vi "InitConfigutation.vi"(8 "error in":errorcluster) -> (0 "error out":errorcluster)   [LabVIEW 2013]
uses:
  <vilib>/Utility/config.llb/Read Key (U32).vi
  <vilib>/Utility/config.llb/Read Key (String).vi
  GlobalVariables/ValveParameters.vi
  GlobalVariables/CaptParameters.vi
  GlobalVariables/SystemParameters.vi
  <vilib>/Utility/config.llb/NI_LVConfig.lvlib
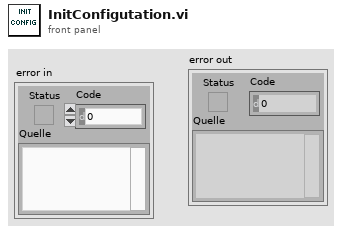
[diagram p1: front panel]
types:
  T1 = cluster{"Mode":enum16{"RTU", "ASCII"}, "Slave Address":u8}
  T2 = typedef "NI_LVConfig.lvlib/Config Data RefNum.ctl" = refnum<k1>
  T3 = cluster{"value":u32, "value":u32, "value":u32, "value":u32, "value":u32}
  T4 = cluster{"value":u32, "value":u32, "value":u32, "value":u32, "value":u32, "value":string, "Serial Parameters":cluster{"Mode":enum16{"RTU", "ASCII"}, "Slave Address":u8}, "value":u32, cluster{"value":u32, "value":u32, "value":u32, "value":u32, "value":u32}}
  T5 = cluster{"value":u32, "value":u32, "value":u32, "value":u32, "value":u32, "value":string, "value":u32, "Serial Parameters":cluster{"Mode":enum16{"RTU", "ASCII"}, "Slave Address":u8}, "value":u32}
  T6 = cluster{"value":string, "value":string, "value":string, "value":string}
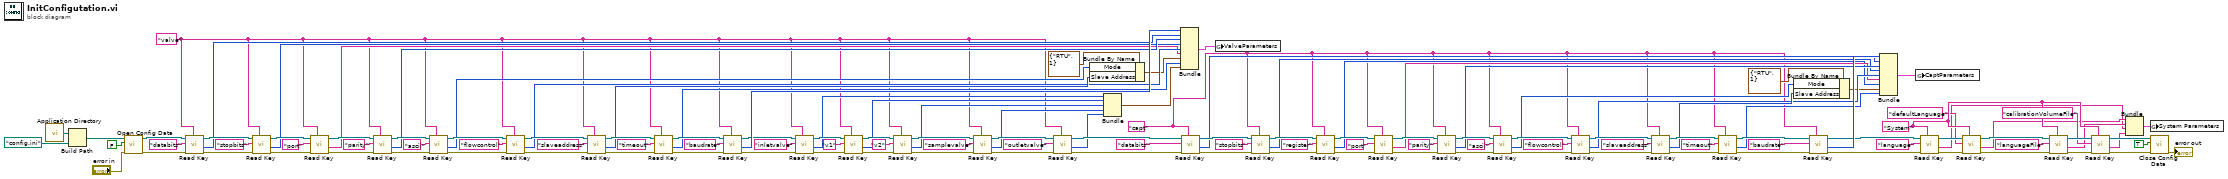
[diagram p0: block diagram]
diagram:
  w34 = "System" ("section")
  w45 = "capt" ("section")
  w6 = "valve" ("section")
  n1 = call <vilib>:"Application Directory.vi"() -> ("Application Directory"=w127:path)
  n2 = Build Path(base path=w127, name or relative path=path "config.ini" ("default name")) -> (appended path=w129:path)
  n3 = call <vilib>:"Open Config Data.vi"("error in (no error)"="error in", "create file if necessary (T)"=FALSE ("create file if necessary? (T)"), "configuration file path"=w129) -> ("error out"=w60:errorcluster, "refnum"=w59:T2)  [unwired: 6 in, 1 out]
  n4 = call-poly <vilib>:"Read Key.vi"("section"=w6, "error in (no error)"=w60, "key"="databits", "refnum"=w59) -> ("error out"=w63:errorcluster, "value"=w55:u32, "refnum out"=w62:T2)  [unwired: 4 in, 1 out]
  n5 = call-poly <vilib>:"Read Key.vi"("section"=w6, "error in (no error)"=w63, "key"="stopbits", "refnum"=w62) -> ("error out"=w61:errorcluster, "value"=w54:u32, "refnum out"=w58:T2)  [unwired: 4 in, 1 out]
  n6 = call-poly <vilib>:"Read Key.vi"("section"=w6, "error in (no error)"=w61, "key"="port", "refnum"=w58) -> ("error out"=w120:errorcluster, "value"=w100:string, "refnum out"=w119:T2)  [unwired: 4 in, 1 out]
  n7 = call-poly <vilib>:"Read Key.vi"("section"=w6, "error in (no error)"=w120, "key"="parity", "refnum"=w119) -> ("error out"=w117:errorcluster, "value"=w102:u32, "refnum out"=w114:T2)  [unwired: 4 in, 1 out]
  n8 = call-poly <vilib>:"Read Key.vi"("section"=w6, "error in (no error)"=w117, "key"="ascii", "refnum"=w114) -> ("error out"=w116:errorcluster, "value"=w107:u32, "refnum out"=w115:T2)  [unwired: 4 in, 1 out]
  n9 = call-poly <vilib>:"Read Key.vi"("section"=w6, "error in (no error)"=w116, "key"="flowcontrol", "refnum"=w115) -> ("error out"=w112:errorcluster, "value"=w101:u32, "refnum out"=w109:T2)  [unwired: 4 in, 1 out]
  n10 = call-poly <vilib>:"Read Key.vi"("section"=w6, "error in (no error)"=w112, "key"="slaveaddress", "refnum"=w109) -> ("error out"=w111:errorcluster, "value"=w106:u32, "refnum out"=w110:T2)  [unwired: 4 in, 1 out]
  n11 = call-poly <vilib>:"Read Key.vi"("section"=w6, "error in (no error)"=w111, "key"="timeout", "refnum"=w110) -> ("error out"=w124:errorcluster, "value"=w98:u32, "refnum out"=w125:T2)  [unwired: 4 in, 1 out]
  n12 = call-poly <vilib>:"Read Key.vi"("section"=w6, "error in (no error)"=w124, "key"="baudrate", "refnum"=w125) -> ("error out"=w23:errorcluster, "value"=w103:u32, "refnum out"=w13:T2)  [unwired: 4 in, 1 out]
  n13 = call-poly <vilib>:"Read Key.vi"("section"=w6, "error in (no error)"=w23, "key"="inletvalve", "refnum"=w13) -> ("error out"=w24:errorcluster, "value"=w11:u32, "refnum out"=w14:T2)  [unwired: 4 in, 1 out]
  n14 = call-poly <vilib>:"Read Key.vi"("section"=w6, "error in (no error)"=w24, "key"="v1", "refnum"=w14) -> ("error out"=w22:errorcluster, "value"=w10:u32, "refnum out"=w15:T2)  [unwired: 4 in, 1 out]
  n15 = call-poly <vilib>:"Read Key.vi"("section"=w6, "error in (no error)"=w22, "key"="v2", "refnum"=w15) -> ("error out"=w21:errorcluster, "value"=w9:u32, "refnum out"=w16:T2)  [unwired: 4 in, 1 out]
  n16 = call-poly <vilib>:"Read Key.vi"("section"=w6, "error in (no error)"=w21, "key"="samplevalve", "refnum"=w16) -> ("error out"=w20:errorcluster, "value"=w8:u32, "refnum out"=w17:T2)  [unwired: 4 in, 1 out]
  n17 = call-poly <vilib>:"Read Key.vi"("section"=w6, "error in (no error)"=w20, "key"="outletvalve", "refnum"=w17) -> ("error out"=w19:errorcluster, "value"=w7:u32, "refnum out"=w18:T2)  [unwired: 4 in, 1 out]
  n18 = Bundle By Name(cluster=T1 {"Mode"=enum."RTU", "Slave Address"=1} ("Serial Parameters"), "Mode"=w107, "Slave Address"=w106) -> (w99:T1)
  n19 = Bundle("value"=w11, "value"=w10, "value"=w9, "value"=w8, "value"=w7) -> (w12:T3)  [unwired: 1 in]
  n20 = Bundle("value"=w103, "value"=w55, "value"=w102, "value"=w54, "value"=w101, "value"=w100, "Serial Parameters"=w99, "value"=w98, w12) -> (w104:T4)  [unwired: 1 in]
  n21 = call-poly <vilib>:"Read Key.vi"("section"=w45, "error in (no error)"=w19, "key"="databits", "refnum"=w18) -> ("error out"=w53:errorcluster, "value"=w47:u32, "refnum out"=w52:T2)  [unwired: 4 in, 1 out]
  n22 = global write "ValveParameters.vi" "ValveParameters"(w104) -> ()
  n23 = call-poly <vilib>:"Read Key.vi"("section"=w45, "error in (no error)"=w53, "key"="stopbits", "refnum"=w52) -> ("error out"=w48:errorcluster, "value"=w46:u32, "refnum out"=w49:T2)  [unwired: 4 in, 1 out]
  n24 = call-poly <vilib>:"Read Key.vi"("section"=w45, "error in (no error)"=w48, "key"="register", "refnum"=w49) -> ("error out"=w67:errorcluster, "value"=w65:u32, "refnum out"=w66:T2)  [unwired: 4 in, 1 out]
  n25 = call-poly <vilib>:"Read Key.vi"("section"=w45, "error in (no error)"=w67, "key"="port", "refnum"=w66) -> ("error out"=w91:errorcluster, "value"=w72:string, "refnum out"=w90:T2)  [unwired: 4 in, 1 out]
  n26 = call-poly <vilib>:"Read Key.vi"("section"=w45, "error in (no error)"=w91, "key"="parity", "refnum"=w90) -> ("error out"=w88:errorcluster, "value"=w74:u32, "refnum out"=w85:T2)  [unwired: 4 in, 1 out]
  n27 = call-poly <vilib>:"Read Key.vi"("section"=w45, "error in (no error)"=w88, "key"="ascii", "refnum"=w85) -> ("error out"=w87:errorcluster, "value"=w78:u32, "refnum out"=w86:T2)  [unwired: 4 in, 1 out]
  n28 = call-poly <vilib>:"Read Key.vi"("section"=w45, "error in (no error)"=w87, "key"="flowcontrol", "refnum"=w86) -> ("error out"=w83:errorcluster, "value"=w73:u32, "refnum out"=w80:T2)  [unwired: 4 in, 1 out]
  n29 = call-poly <vilib>:"Read Key.vi"("section"=w45, "error in (no error)"=w83, "key"="slaveaddress", "refnum"=w80) -> ("error out"=w82:errorcluster, "value"=w77:u32, "refnum out"=w81:T2)  [unwired: 4 in, 1 out]
  n30 = call-poly <vilib>:"Read Key.vi"("section"=w45, "error in (no error)"=w82, "key"="timeout", "refnum"=w81) -> ("error out"=w94:errorcluster, "value"=w70:u32, "refnum out"=w95:T2)  [unwired: 4 in, 1 out]
  n31 = Bundle By Name(cluster=T1 {"Mode"=enum."RTU", "Slave Address"=1} ("Serial Parameters"), "Mode"=w78, "Slave Address"=w77) -> (w71:T1)
  n32 = call-poly <vilib>:"Read Key.vi"("section"=w45, "error in (no error)"=w94, "key"="baudrate", "refnum"=w95) -> ("error out"=w44:errorcluster, "value"=w75:u32, "refnum out"=w43:T2)  [unwired: 4 in, 1 out]
  n33 = Bundle("value"=w75, "value"=w47, "value"=w74, "value"=w46, "value"=w73, "value"=w72, "value"=w65, "Serial Parameters"=w71, "value"=w70) -> (w68:T5)  [unwired: 1 in]
  n34 = global write "CaptParameters.vi" "CaptParameters"(w68) -> ()
  n35 = call-poly <vilib>:"Read Key.vi"("section"=w34, "error in (no error)"=w44, "key"="language" ("section"), "refnum"=w43) -> ("error out"=w35:errorcluster, "value"=w27:string, "refnum out"=w42:T2)  [unwired: 4 in, 1 out]
  n36 = call-poly <vilib>:"Read Key.vi"("section"=w34, "error in (no error)"=w35, "key"="defaultLanguage" ("section"), "refnum"=w42) -> ("error out"=w36:errorcluster, "value"=w29:string, "refnum out"=w41:T2)  [unwired: 4 in, 1 out]
  n37 = call-poly <vilib>:"Read Key.vi"("section"=w34, "error in (no error)"=w36, "key"="languageFile" ("section"), "refnum"=w41) -> ("error out"=w37:errorcluster, "value"=w28:string, "refnum out"=w40:T2)  [unwired: 4 in, 1 out]
  n38 = call-poly <vilib>:"Read Key.vi"("section"=w34, "error in (no error)"=w37, "key"="calibrationVolumeFile" ("section"), "refnum"=w40) -> ("error out"=w38:errorcluster, "value"=w26:string, "refnum out"=w39:T2)  [unwired: 4 in, 1 out]
  n39 = Bundle("value"=w29, "value"=w28, "value"=w27, "value"=w26) -> (w25:T6)  [unwired: 1 in]
  n40 = global write "SystemParameters.vi" "System Parameters"(w25) -> ()
  n41 = call <vilib>:"Close Config Data.vi"("error in (no error)"=w38, "write file if changed (T)"=TRUE ("write configuration file? (T)"), "refnum"=w39) -> ("error out"=→"error out":errorcluster)  [unwired: 8 out]
